vi "Pneumatics_Open.vi"(8 "error in":errorcluster) -> (0 "error out":errorcluster)   [LabVIEW 2020]
uses:
  <vilib>/Rock Robotics/WPI/Solenoid/WPI_SolenoidChannel.ctl
  <vilib>/Rock Robotics/SystemInterfaces/DIO/FPGA_DIOChannel.ctl
  <vilib>/Rock Robotics/WPI/Utilities/WPI_GetSetVariantRefNum.vi
  <vilib>/Rock Robotics/WPI/Solenoid/WPI_SolenoidOpenSingle.vi
  <vilib>/Rock Robotics/WPI/Solenoid/WPI_SolenoidOpenDouble.vi
  <vilib>/Rock Robotics/WPI/Switch/WPI_SwitchOpenLimit.vi
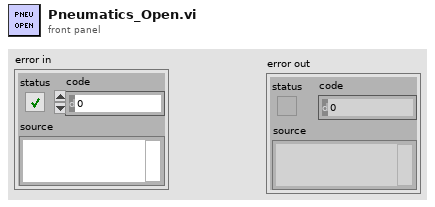
[diagram p1: front panel]
types:
  T1 = typedef "FPGA_DIOChannel.ctl" = enum8{"DIO 0", "DIO 1", "DIO 2", "DIO 3", "DIO 4", "DIO 5", "DIO 6", "DIO 7", "DIO 8", "DIO 9", "DIO MXP 0", "DIO MXP 1", "DIO MXP 2", "DIO MXP 3", "DIO MXP 4", "DIO MXP 5", "DIO MXP 6", "DIO MXP 7", "DIO MXP 8", "DIO MXP 9", "DIO MXP 10", "DIO MXP 11", "DIO MXP 12", "DIO MXP 13", "DIO MXP 14", "DIO MXP 15", "SPI Port CS1", "SPI Port CS2", "SPI Port CS3", "SPI Port MISO", "SPI Port MOSI", "Invalid"}
  T2 = typedef "WPI_SolenoidChannel.ctl" = enum8{"Solenoid 0", "Solenoid 1", "Solenoid 2", "Solenoid 3", "Solenoid 4", "Solenoid 5", "Solenoid 6", "Solenoid 7", "Solenoid 8", "Solenoid 9", "Solenoid 10", "Solenoid 11", "Solenoid 12", "Solenoid 13", "Solenoid 14", "Solenoid 15", "Invalid"}
  T3 = typedef "WPI_CompressorDevRef.ctl" = cluster{"DevStatus":errorcluster, "Pneumatics Control Module":u8}
  T4 = typedef "WPI_SwitchDevRef.ctl" = cluster{"DevStatus":errorcluster, "DIO Channel":T1, "CntIndex":T5, "Normally Closed":bool}
  T5 = typedef "FPGA_CounterCtrSystemIndex.ctl" = enum8{"Ctr 0", "Ctr 1", "Ctr 2", "Ctr 3", "Ctr 4", "Ctr 5", "Ctr 6", "Ctr 7", "Invalid"}
  T6 = typedef "WPI_SolenoidDevRef.ctl" = cluster{"DevStatus":errorcluster, "Pneumatics Control Module":u8, "Forward Solenoid Channel":T2, "Reverse Solenoid Channel":T2}
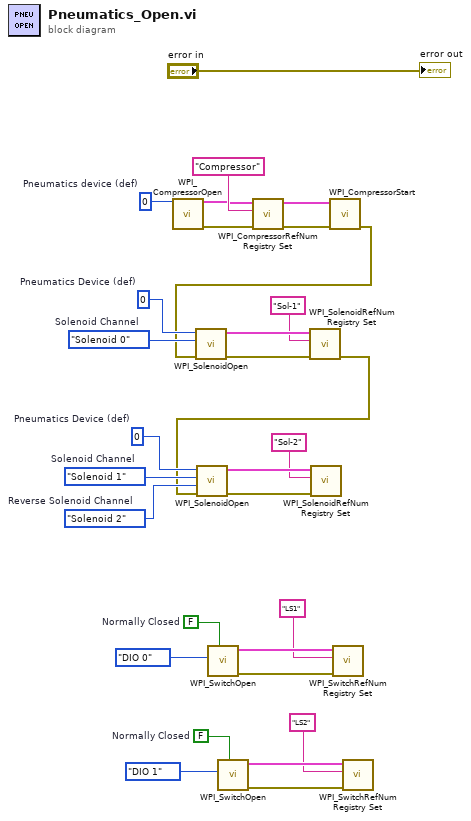
[diagram p0: block diagram]
diagram:
  w3 = FALSE  # Normally Closed
  w8 = FALSE  # Normally Closed
  w13 = WPI_SolenoidChannel."Solenoid 2"  # Reverse Solenoid Channel
  w14 = WPI_SolenoidChannel."Solenoid 1"  # Solenoid Channel
  w15 = u8 0  # Pneumatics Device (def)
  w19 = WPI_SolenoidChannel."Solenoid 0"  # Solenoid Channel
  w20 = u8 0  # Pneumatics Device (def)
  w29 = u8 0  # Pneumatics device (def)
  n1 = call <vilib>:"WPI_CompressorOpen.vi"("Pneumatics device (def)"=w29) -> ("CompressorDevRef"=w24:T3, "error out"=w27:errorcluster)  [unwired: 13 in]
  n2 = call-poly <vilib>:"WPI_SwitchOpen.vi"("Normally Closed"=w8, "DIO Channel"=FPGA_DIOChannel."DIO 0") -> ("error out"=w9:errorcluster, "SwitchDevRef"=w10:T4)  [unwired: 8 in]
  n3 = call-poly <vilib>:"WPI_SwitchOpen.vi"("Normally Closed"=w3, "DIO Channel"=FPGA_DIOChannel."DIO 1") -> ("error out"=w4:errorcluster, "SwitchDevRef"=w5:T4)  [unwired: 8 in]
  n4 = call <vilib>:"WPI_CompressorRefNum Registry Set.vi"("error in (no error)"=w27, "refnum name"="Compressor", "CompressorDevRef"=w24) -> ("error out"=w25:errorcluster, "CompressorDevRef"=w26:T3)  [unwired: 7 in]
  n5 = call <vilib>:"WPI_CompressorStart.vi"("error in (no error)"=w25, "CompressorDevRef"=w26) -> ("error out"=w12:errorcluster)  [unwired: 8 in, 1 out]
  n6 = call-poly <vilib>:"WPI_SolenoidOpen.vi"("error in (no error)"=w12, "Solenoid Channel"=w19, "Pneumatics Device (def)"=w20) -> ("error out"=w22:errorcluster, "SolenoidDevRef"=w23:T6)  [unwired: 7 in]
  n7 = call <vilib>:"WPI_SolenoidRefNum Registry Set.vi"("error in (no error)"=w22, "refnum name"="Sol-1", "SolenoidDevRef"=w23) -> ("error out"=w11:errorcluster)  [unwired: 7 in, 1 out]
  n8 = call-poly <vilib>:"WPI_SolenoidOpen.vi"("error in (no error)"=w11, "Reverse Solenoid Channel"=w13, "Forward Solenoid Channel"=w14, "Pneumatics Device (def)"=w15) -> ("error out"=w17:errorcluster, "SolenoidDevRef"=w18:T6)  [unwired: 6 in]
  n9 = call <vilib>:"WPI_SolenoidRefNum Registry Set.vi"("error in (no error)"=w17, "refnum name"="Sol-2", "SolenoidDevRef"=w18) -> ()  [unwired: 7 in, 2 out]
  n10 = call <vilib>:"WPI_SwitchRefNum Registry Set.vi"("error in (no error)"=w9, "refnum name"="LS1", "SwitchDevRef"=w10) -> ()  [unwired: 7 in, 2 out]
  n11 = call <vilib>:"WPI_SwitchRefNum Registry Set.vi"("error in (no error)"=w4, "refnum name"="LS2", "SwitchDevRef"=w5) -> ()  [unwired: 7 in, 2 out]
  "error out" <- "error in"
